vi "GWD_Query.vi"(0 "System no.":i32=1 min=1 max=4 step=1, 2 "Query axis":string, 5 "error in":errorcluster, 6 "Xo":i32, 7 "N":i32=10, 8 "Nmax":i32=64) -> (14 "Waveform points":dbl[](array[numeric]) format="%.6f", 15 "GWD? string":string, 19 "error out":errorcluster)   [LabVIEW 2020]
doc: "Returns N waveform sequence points. Nmax is the maximum number of points that can be read at once. If N > Nmax, then the VI will query GWD? more than once to read all N values. \n\nC-413: Query axis is identical with wave table number, which can be 1 to 8 . Nmax must be less than or equal to the length of the defined wave. Xo must be greater than zero.\n\nC-886: Query axis is identical with wave table number. Nmax must be less than or equal to the length of the defined wave. Xo must be greater than zero.\n\nC-887: Query axis is identical with wave table number, which can be 1 to 100. Nmax must be less than or equal to the length of the defined wave. Xo must be greater than zero.\n\nC-891: Query axis is identical with wave table number, which can be 1 to 40. Nmax must be less than or equal to the length of the defined wave. Xo must be greater than zero. The GWD? command is present for compatibility reasons only. The response to GWD? only contains the header, but no waveform values.\n\nE-516: Nmax = 5, N can be 8192 maximum\n\nE-517, E-518: Query axis is identical with wave table number, which can be 1 to 3. Nmax must be less than or equal to the length of the defined wave. Xo must be greater than zero. The response to GWD? does not contain any offset to the wave generator output set with WOS.\n\nE-709: Query axis is identical with wave table number, which can be 1 to 4. Nmax must be less than or equal to the length of the defined wave. The recommended Nmax value is 1000. For larger values it might be necessary to increase the timeout value in E709_Configuration_Setup.vi. Xo must be greater than zero.\n\nE-710: Query axis is identical with wave table number. Nmax must be less than the length of the defined wave.\n\nE-712: Query axis is identical with wave table number, which can be 1 to 90. Nmax must be less than or equal to the length of the defined wave. Xo must be greater than zero.\n\nE-725: Query axis is identical with wave table number, which can be 1 to 30. Nmax must be less than or equal to the length of the defined wave. Xo must be greater than zero.\n\nE-727: Query axis is identical with wave table number, which can be 1 to 40. Nmax must be less than or equal to the length of the defined wave. Xo must be greater than zero.\n\nE-753: Query axis is identical with wave table number, which can be 1 to 10. Nmax must be less than or equal to the length of the defined wave. Xo must be greater than zero.\n\nE-754: Query axis is identical with wave table number, which can be 1 to 10. Nmax must be less than or equal to the length of the defined wave. Xo must be greater than zero.\n\nE-761: Query axis is identical with wave table number, which can be 1 to 4. Nmax must be less than the length of the defined wave. The content of a wave table is not completely erased when a new waveform is written to this table. Only the number of points given by the new waveform is written beginning with the first point in the table, but any subsequent data points will keep the old values from the former waveform. This affects only the response to the GWD? query and not the wave generator output which will only send the new waveform points."
uses:
  Syntax.ctl
  Global1.vi
panel:
  # "Returns N waveform sequence points. Nmax is the maximum number of points that can be read at once. If N > Nmax, then the VI will query GWD? more than once to read all N values."
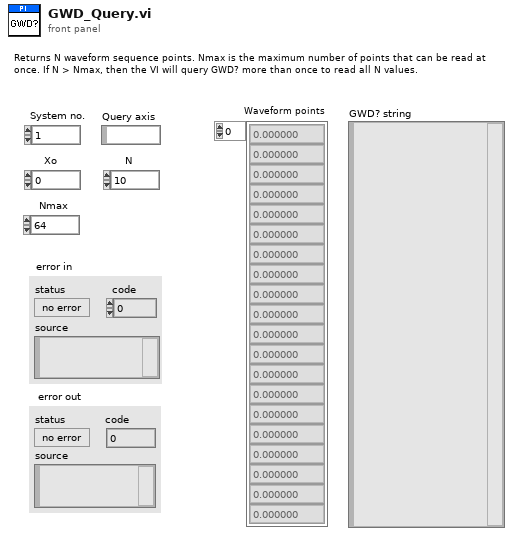
[diagram p1: front panel]
types:
  T1 = typedef "Syntax.ctl" = enum16{"GCS 1.0", "GCS 2.0", "GCS 3.0"}
  T2 = cluster{"Read (F)/Write":bool, "Path":path, "Datastream":string, "ArrayName":string}
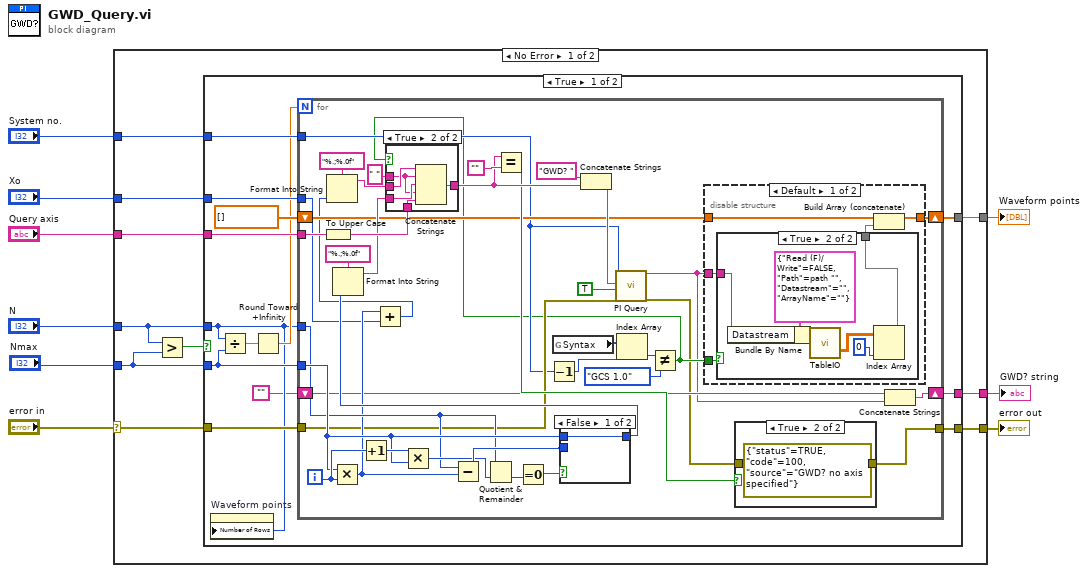
[diagram p0: block diagram]
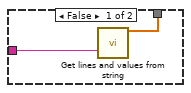
[diagram p2: hidden frame]
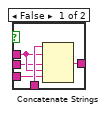
[diagram p4: hidden frame]
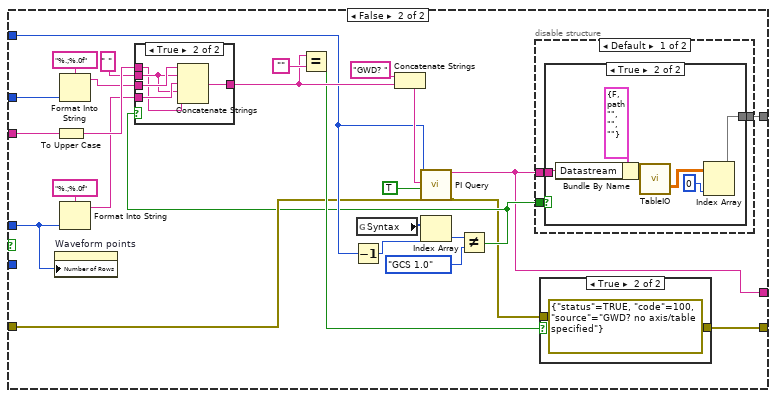
[diagram p7: hidden frame]
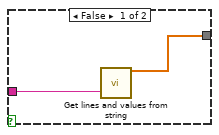
[diagram p8: hidden frame]
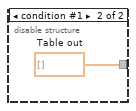
[diagram p9: hidden frame]
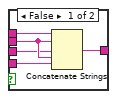
[diagram p10: hidden frame]
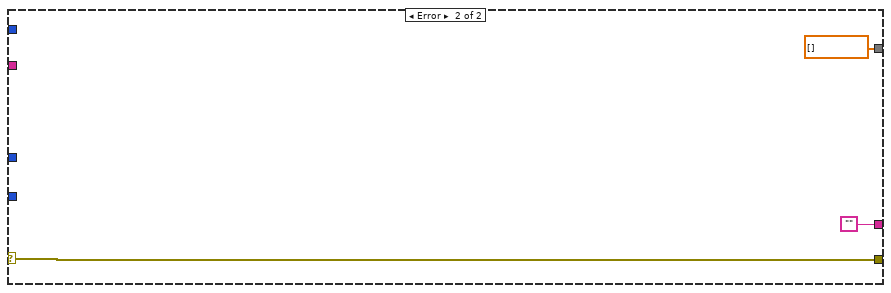
[diagram p12: hidden frame]
diagram:
  n1 = case shown="No Error" "error in" {
    selector: "error in" -> [w10 w150]
    tunnel: "System no." -> [w19 _]
    tunnel: "Query axis" -> [w18 _]
    tunnel: "Xo" -> [w17 _]
    tunnel: [w16 w150] -> w6
    tunnel: "N" -> [w15 _]
    tunnel: [w14 dbl[] []] -> w4
    tunnel: "Nmax" -> [w12 _]
    tunnel: [w11 ""] -> w2
    frame No Error {
      n2 = Greater?(x=w15, y=w12) -> (0:w13:bool)
      n3 = case shown="True" w13 {
        tunnel: w19 -> [w32 w105]
        tunnel: w18 -> [w31 w122]
        tunnel: w17 -> [w30 w117]
        tunnel: [w29 w112] -> w16
        tunnel: w15 -> [w22 w111]
        tunnel: [w27 w109] -> w14
        tunnel: w10 -> [w28 w104]
        tunnel: w12 -> [w23 _]
        tunnel: [w21 w101] -> w11
        frame True {
          n4 = property on="Waveform points" class="Arr (strict)"("Number of Rows"=w22) -> ()  [unwired: 2 in, 2 out]
          n5 = Divide(x=w22, y=w23) -> (x/y=w25:dbl)
          n6 = Round Toward +Infinity(x=w25) -> (ceil(x): smallest int >= x=w24:dbl)
          n7 = for {
            N: w24 -> [_]
            tunnel: w32 -> [w39]
            tunnel: w31 -> [w68]
            tunnel: w30 -> [w45]
            tunnel: [w59] -> w29
            tunnel: w22 -> [w47]
            tunnel: w28 -> [w43]
            shift-right: [w57] -> w27
            shift-left: dbl[] [] -> [w56]
            tunnel: w23 -> [w49]
            shift-right: [w37] -> w21
            shift-left: "" -> [w36]
            i -> [w55]
            n8 = To Upper Case(1:w68) -> (0:w67:string)
            n9 = Multiply(x=w49, y=w55) -> (x*y=w46:i32)
            n10 = Increment(x=w55) -> (x+1=w54:i32)
            n11 = Add(x=w46, y=w45) -> (x+y=w44:i32)
            n12 = Format Into String(format string="%.;%.0f" ("Format String"), w44) -> (resulting string=w63:string)  [unwired: 2 in, 1 out]
            n13 = Multiply(x=w54, y=w49) -> (x*y=w48:i32)
            n14 = Subtract(x=w47, y=w46) -> (x-y=w50:i32)
            n15 = Quotient & Remainder(x=w47, y=w48) -> (floor(x/y)=w53:i32)  [unwired: 1 out]
            n16 = Equal To 0?(x=w53) -> (x = 0?=w52:bool)
            n17 = Decrement(x=w39) -> (x-1=w41:i32)
            n18 = global read "Global1.vi" "Syntax"() -> (w40:T1[])
            n19 = case shown="False" w52 {
              tunnel: w49 -> [w96 _]
              tunnel: [w96 w97] -> w51
              tunnel: w50 -> [_ w97]
              frame False {
              }
              frame True {
              }
            }
            n20 = Format Into String(format string="%.;%.0f" ("Format String"), w51) -> (resulting string=w62:string)  [unwired: 2 in, 1 out]
            n21 = Index Array(array=w40, index=w41) -> (element=w42:T1)
            n22 = Not Equal?(x=w42, y=Syntax."GCS 1.0") -> (x != y?=w38:bool)
            n23 = case shown="True" w38 {
              tunnel: w67 -> [w90 w91]
              tunnel: " " -> [w89 w92]
              tunnel: w63 -> [w88 w94]
              tunnel: w62 -> [w87 w93]
              tunnel: [w86 w95] -> w61
              frame False {
                n24 = Concatenate Strings(w90, w89, w88, w89, w87) -> (w86:string)
              }
              frame True {
                n25 = Concatenate Strings(w94, w92, w93, w92, w91) -> (w95:string)
              }
            }
            n26 = Equal?(x=w61, y="" ("x")) -> (x = y?=w60:bool)
            n27 = Concatenate Strings("GWD? ", w61) -> (w70:string)
            n28 = call "PI Query.vi"("System no."=w39, "String to send"=w70, "Attach termination char.?"=TRUE ("Attach Linefeed?"), "error in"=w43) -> ("String read"=w34:string, "error out"=w35:errorcluster)  [unwired: 3 in, 11 out]
            n29 = disable-structure shown="Default" {
              disable-tunnel: [w76 w85] -> w57
              disable-tunnel: w56 -> [w75 w85]
              disable-tunnel: w34 -> [w74 _]
              disable-tunnel: w38 -> [w73 _]
              frame condition #0 (active) {
                n30 = case shown="True" w73 {
                  tunnel: w74 -> [w78 w81]
                  tunnel: [w77 w79] -> w72
                  frame False {
                    n31 = call "Get lines and values from string.vi"("Input string"=w78) -> ("Numerical values"=w77:dbl[])  [unwired: 4 in, 14 out]
                  }
                  frame True {
                    n32 = Bundle By Name(cluster=T2 {"Read (F)/Write"=FALSE, "Path"=path "", "Datastream"="", "ArrayName"=""} ("IOSource"), "Datastream"=w81) -> (w82:T2)
                    n33 = call "TableIO.vi"("IOSource"=w82) -> ("Table out"=w84:dbl[][])  [unwired: 5 in, 13 out]
                    n34 = Index Array(array=w84, index (col)=0 ("index (row)")) -> (element=w79:dbl[])  [unwired: 1 in]
                  }
                }
                n35 = Build Array (concatenate)(w75, w72) -> (w76:dbl[])
              }
              frame condition #1 {
              }
            }
            n36 = case shown="True" w60 {
              tunnel: [w98 errorcluster {"status"=TRUE, "code"=100, "source"="GWD? no axis specified"} ("error out")] -> w59
              tunnel: w35 -> [w98 _]
              frame False {
              }
              frame True {
              }
            }
            n37 = Concatenate Strings(w36, w34) -> (w37:string)
          }
        }
        frame False {
          n38 = property on="Waveform points" class="Arr (strict)"("Number of Rows"=w111) -> ()  [unwired: 2 in, 2 out]
          n39 = To Upper Case(1:w122) -> (0:w121:string)
          n40 = Format Into String(format string="%.;%.0f" ("Format String"), w117) -> (resulting string=w116:string)  [unwired: 2 in, 1 out]
          n41 = Format Into String(format string="%.;%.0f" ("Format String"), w111) -> (resulting string=w115:string)  [unwired: 2 in, 1 out]
          n42 = Decrement(x=w105) -> (x-1=w107:i32)
          n43 = global read "Global1.vi" "Syntax"() -> (w106:T1[])
          n44 = Index Array(array=w106, index=w107) -> (element=w108:T1)
          n45 = Not Equal?(x=w108, y=Syntax."GCS 1.0") -> (x != y?=w103:bool)
          n46 = case shown="True" w103 {
            tunnel: w121 -> [w142 w143]
            tunnel: " " -> [w141 w144]
            tunnel: w116 -> [w140 w146]
            tunnel: w115 -> [w139 w145]
            tunnel: [w138 w147] -> w114
            frame False {
              n47 = Concatenate Strings(w142, w141, w140, w141, w139) -> (w138:string)
            }
            frame True {
              n48 = Concatenate Strings(w146, w144, w145, w144, w143) -> (w147:string)
            }
          }
          n49 = Equal?(x=w114, y="" ("x")) -> (x = y?=w113:bool)
          n50 = Concatenate Strings("GWD? ", w114) -> (w124:string)
          n51 = call "PI Query.vi"("System no."=w105, "String to send"=w124, "Attach termination char.?"=TRUE ("Attach Linefeed?"), "error in"=w104) -> ("String read"=w101:string, "error out"=w102:errorcluster)  [unwired: 3 in, 11 out]
          n52 = disable-structure shown="Default" {
            disable-tunnel: [w128 w137] -> w109
            disable-tunnel: w103 -> [w127 _]
            disable-tunnel: w101 -> [w126 _]
            frame condition #0 (active) {
              n53 = case shown="True" w127 {
                tunnel: w126 -> [w130 w133]
                tunnel: [w129 w132] -> w128
                frame False {
                  n54 = call "Get lines and values from string.vi"("Input string"=w130) -> ("Numerical values"=w129:dbl[])  [unwired: 4 in, 14 out]
                }
                frame True {
                  n55 = Bundle By Name(cluster=T2 {"Read (F)/Write"=FALSE, "Path"=path "", "Datastream"="", "ArrayName"=""} ("IOSource"), "Datastream"=w133) -> (w134:T2)
                  n56 = call "TableIO.vi"("IOSource"=w134) -> ("Table out"=w136:dbl[][])  [unwired: 5 in, 13 out]
                  n57 = Index Array(array=w136, index (col)=0 ("index (row)")) -> (element=w132:dbl[])  [unwired: 1 in]
                }
              }
            }
            frame condition #1 {
              w137 = dbl[] []  # Table out
            }
          }
          n58 = case shown="True" w113 {
            tunnel: [w148 errorcluster {"status"=TRUE, "code"=100, "source"="GWD? no axis/table specified"} ("error out")] -> w112
            tunnel: w102 -> [w148 _]
            frame False {
            }
            frame True {
            }
          }
        }
      }
    }
    frame Error {
    }
  }
  "error out" <- w6
  "Waveform points" <- w4
  "GWD? string" <- w2
